vi "data_log_count_500.vi"(8 "error in (no error)":errorcluster, 10 "All data":string[](array[string]), 11 "file path (dialog if empty)":path=path "E:/Work/NI Vision/Tata_ficoso Data Logging Software/XBA/XBA ORVM V2/Data/Previous_Part_data.csv") -> (0 "error out":errorcluster)   [LabVIEW 2017]
uses:
  <vilib>/Utility/file.llb/Write Delimited Spreadsheet (string).vi
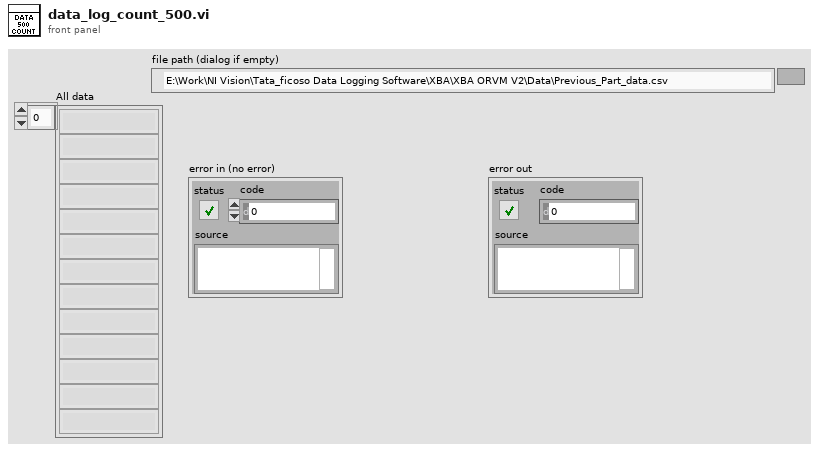
[diagram p1: front panel]
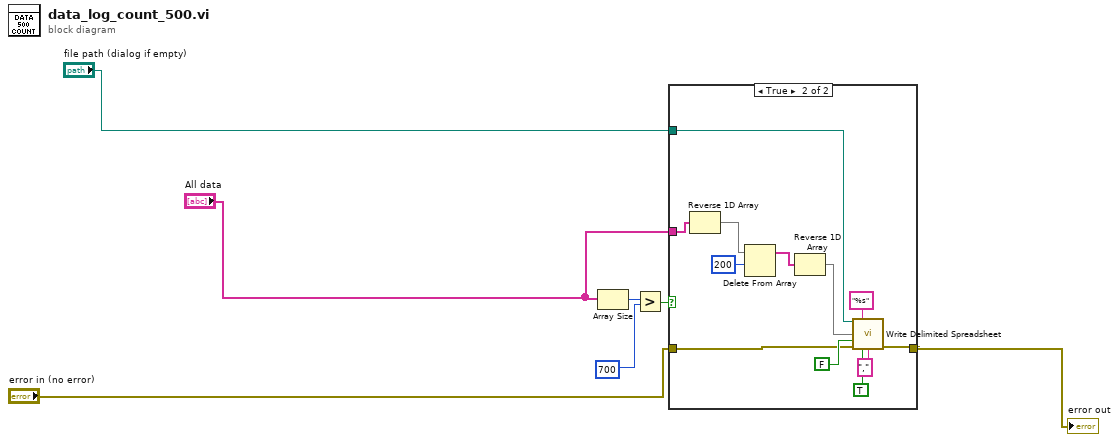
[diagram p0: block diagram]
diagram:
  n1 = Array Size(array="All data") -> (size(s)=w5:i32)
  n2 = Greater?(x=w5, y=700) -> (0:w3:bool)
  n3 = case shown="True" w3 {
    tunnel: "error in (no error)" -> [w8 w17]
    tunnel: [w8 w16] -> w6
    tunnel: "All data" -> [_ w15]
    tunnel: "file path (dialog if empty)" -> [_ w10]
    frame False {
    }
    frame True {
      n4 = Reverse 1D Array(array=w15) -> (reversed array=w13:string[])
      n5 = Delete From Array(array=w13, length=200) -> (array with subset deleted=w12:string[])  [unwired: 1 in, 1 out]
      n6 = Reverse 1D Array(array=w12) -> (reversed array=w11:string[])
      n7 = call-poly <vilib>:"Write Delimited Spreadsheet.vi"("file path (dialog if empty)"=w10, "format (%s)"="%s", "1D data"=w11, "append to file? (new file:F)"=FALSE, "error in (no error)"=w17, "transpose? (no:F)"=TRUE, "delimiter (\\t)"="," ("delimiter (\\t)")) -> ("error out"=w16:errorcluster)  [unwired: 7 in, 1 out]
    }
  }
  "error out" <- w6
